vi "sawtooth waveform generation.vi"() -> ()   [LabVIEW 2025]
panel:
  out "Waveform Graph":dynamicdata(graph)
  in  "phase":dbl
  in  "offset":dbl
  in  "frequency":dbl
  in  "amplitude":dbl
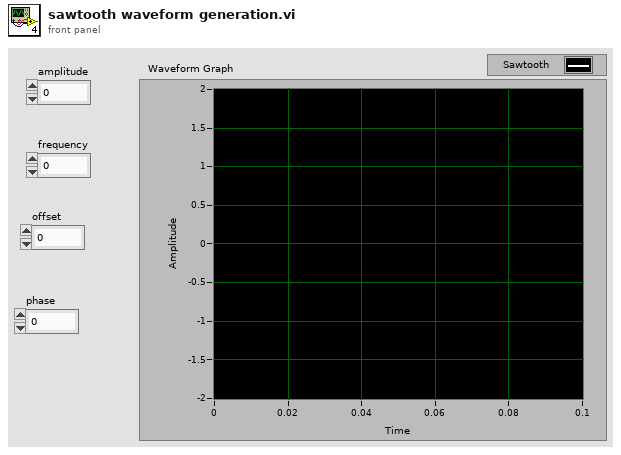
[diagram p1: front panel]
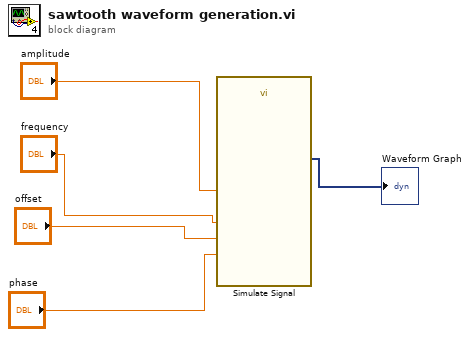
[diagram p0: block diagram]
diagram:
  n1 = call "Simulate Signal"("Offset"="offset", "Frequency"="frequency", "Amplitude"="amplitude", "Phase"="phase") -> ("Sawtooth"=→"Waveform Graph":dynamicdata)  [unwired: 10 in, 1 out]
